vi "Fill Maps.vi"(5 "App Ref":refnum<vi>, 11 "DQMH Modules":refnum<vi>[](array[refnum])) -> (2 "map ref out":map{string, refnum<vi>}(c390), 3 "Tree Map out":T1)   [LabVIEW 2019, in "Panther Dashboard.lvlib"]
uses:
  Panther Dashboard.lvlib
  <vilib>/National Instruments/Tree Map/Tree Map Data.ctl
  Event types--enum.ctl
  <vilib>/National Instruments/Tree Map/Tree Map.lvlib
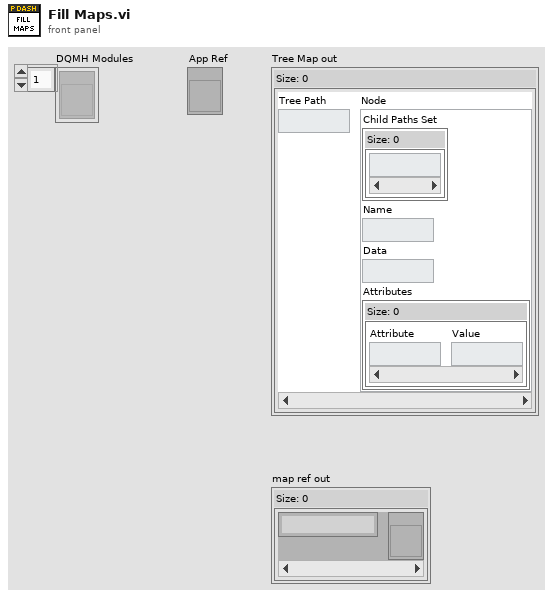
[diagram p1: front panel]
types:
  T1 = typedef "Tree Map.lvlib/Tree Map Data.ctl" = map{string, cluster{"Child Paths Set":set{string}, "Name":string, "Data":string, "Attributes":map{string, string}}}
  T2 = typedef "Panther Dashboard.lvlib/Event types--enum.ctl" = enum16{"Request", "Request and Wait for Reply", "Broadcast"}
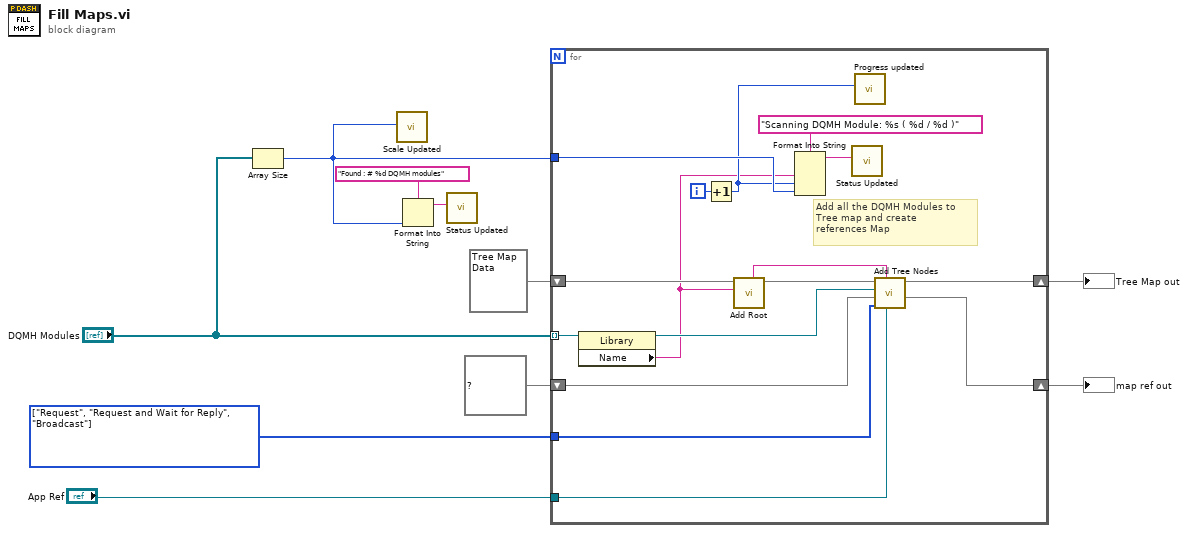
[diagram p0: block diagram]
diagram:
  w8 = T2[] [enum."Request", enum."Request and Wait for Reply", enum."Broadcast"] items=["Request", "Request and Wait for Reply", "Broadcast"] ("Event Types")
  n1 = Array Size(array="DQMH Modules") -> (size(s)=w2:i32)
  n2 = call "Scale Updated.vi"("Scale Max"=w2) -> ()  [unwired: 10 in, 1 out]
  n3 = Format Into String(format string="Found : # %d DQMH modules", w2) -> (resulting string=w7:string)  [unwired: 2 in, 1 out]
  n4 = call "Status Updated.vi"("Status"=w7) -> ()  [unwired: 10 in, 1 out]
  n5 = for {
    shift-right: [w24] -> w3
    shift-left: T1 {} ("Tree Map out") -> [w17]
    shift-right: [w26] -> w10
    shift-left: map{string, refnum<vi>} {} ("References Map") -> [w25]
    tunnel: "DQMH Modules" -> [w16] mode=indexing
    tunnel: w8 -> [w23]
    tunnel: w2 -> [w21]
    tunnel: "App Ref" -> [w15]
    i -> [w22]
    # "Add all the DQMH Modules to\nTree map and create \nreferences Map"
    n6 = property class="Library"(reference=w16) -> (reference out=w12:refnum<vi>, "Name"=w11:string)  [unwired: 1 in, 1 out]
    n7 = Increment(x=w22) -> (x+1=w13:i32)
    n8 = call <vilib>:"Add Root.vi"("New Root Name"=w11, "Tree Map In"=w17) -> ("Tree Map Out"=w18:T1, "Root Path"=w14:string)  [unwired: 8 in]
    n9 = Format Into String(format string="Scanning DQMH Module: %s ( %d / %d )", w11, w13, w21) -> (resulting string=w19:string)  [unwired: 2 in, 1 out]
    n10 = call "Status Updated.vi"("Status"=w19) -> ()  [unwired: 10 in, 1 out]
    n11 = call "Progress updated.vi"("Progress"=w13) -> ()  [unwired: 10 in, 1 out]
    n12 = call "Add Tree Nodes.vi"("App Ref"=w15, "Root path"=w14, "Event Types"=w23, "map ref in"=w25, "DQMH Lib In"=w12, "Tree Map in"=w18) -> ("map ref out"=w26:map{string, refnum<vi>}, "Tree Map out"=w24:T1)  [unwired: 4 in]
  }
  "map ref out" <- w10
  "Tree Map out" <- w3
